vi "8164B Set Power SetPoint (1).vi"(8 "error in":errorcluster, 10 "Power Set Point":dbl=-60.0 format="%#_13g", 11 "KeySight 8164B control in":T1) -> (0 "error out":errorcluster, 3 "KeySight 8164B control out":T1)   [LabVIEW 2018, in "KeySight 8164B LAN InstrLib.lvlib"]
uses:
  KeySight 8164B LAN InstrLib.lvlib
  typedefs/KeySight 8164B control.ctl
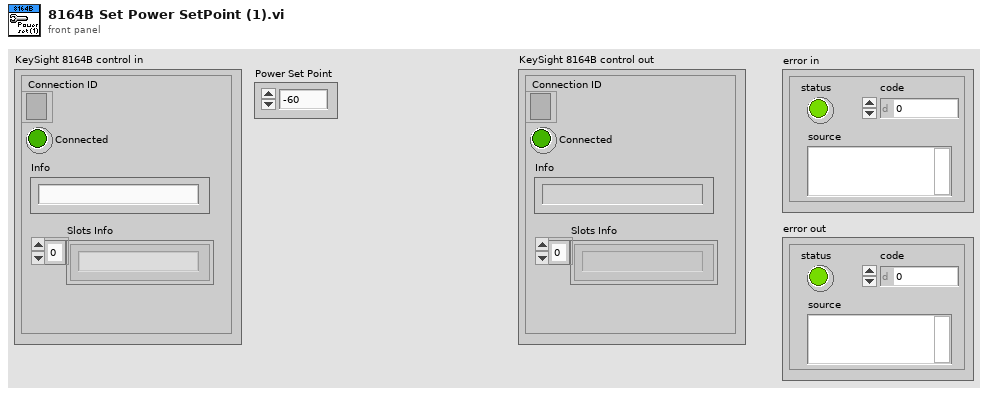
[diagram p1: front panel]
types:
  T1 = typedef "KeySight 8164B LAN InstrLib.lvlib/KeySight 8164B control.ctl" = cluster{"Connection ID":refnum<k5>, "Connected":bool, "Info":string, "Slots Info":string[]}
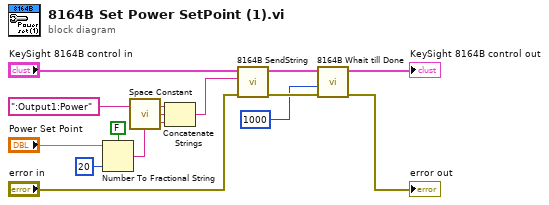
[diagram p0: block diagram]
diagram:
  n1 = Number To Fractional String(use system decimal point (T)=FALSE, number="Power Set Point", precision (6)=i16 20) -> (F-format string=w2:string)  [unwired: 1 in]
  n2 = call <vilib>:"Space Constant.vi"() -> ("String"=w5:string)
  n3 = Concatenate Strings(":Output1:Power", w5, w2) -> (w4:string)
  n4 = call "8164B SendString.vi"("error in"="error in", "CMD"=w4, "KeySight 8164B control in"="KeySight 8164B control in") -> ("error out"=w8:errorcluster, "KeySight 8164B control out"=w10:T1)  [unwired: 7 in]
  n5 = call "8164B Whait till Done.vi"("error in"=w8, "timeout ms"=1000, "KeySight 8164B control in"=w10) -> ("error out"=→"error out":errorcluster, "KeySight 8164B control out"=→"KeySight 8164B control out":T1)  [unwired: 7 in]
